vi "AllowEdgeStartCheck.vi"(0 "reference in":refnum<class "UseCaseDiagramGraph.lvclass">, 1 "EdgeStartNode":refnum<class "AbstractNode.lvclass">, 2 "GraphButton":u32, 5 "error in (no error)":errorcluster) -> (14 "reference out":refnum<class "UseCaseDiagramGraph.lvclass">, 16 "Allowed":bool, 19 "error out":errorcluster)   [LabVIEW 2016, in "UseCaseDiagramGraph.lvclass"]
uses:
  <resource>/Framework/Providers/Open_GDS/UML/UseCaseDiagramGraph_class/UseCaseDiagramGraph.lvclass
  <resource>/Framework/Providers/Open_GDS/UML/AbstractNode_class/AbstractNode.lvclass
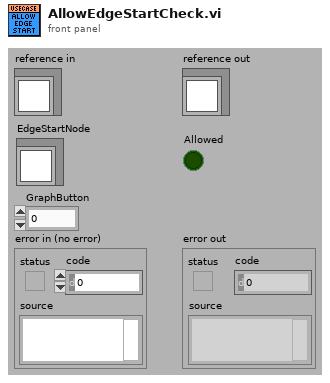
[diagram p1: front panel]
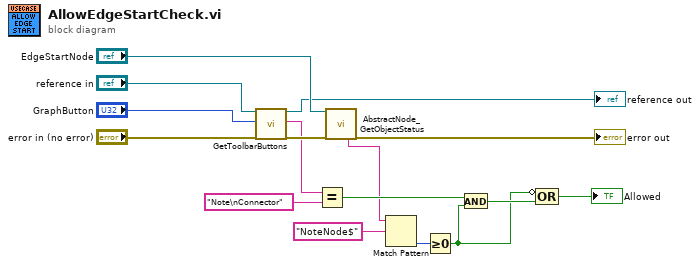
[diagram p0: block diagram]
diagram:
  n1 = call-dynamic "GetToolbarButtons.vi"("reference in"="reference in", "GraphButton"="GraphButton", "error in (no error)"="error in (no error)") -> ("reference out"=→"reference out":refnum<class "UseCaseDiagramGraph.lvclass">, "Text"=w4:string, "error out"=w10:errorcluster)  [unwired: 12 in, 2 out]
  n2 = Equal?(x=w4, y="Note\nConnector" ("Text")) -> (x = y?=w7:bool)
  n3 = call <resource>:"AbstractNode_GetObjectStatus.vi"("reference in"="EdgeStartNode", "error in (no error)"=w10) -> ("Class name"=w6:string, "error out"=→"error out":errorcluster)  [unwired: 16 out]
  n4 = Match Pattern(string=w6, regular expression="NoteNode$") -> (offset past match=w8:i32)  [unwired: 4 out]
  n5 = Greater Or Equal To 0?(x=w8) -> (x >= 0?=w1:bool)
  n6 = And(x=w7, y=w1) -> (x .and. y?=w3:bool)
  n7 = Compound Arithmetic op=OR(invert w1, w3) -> (→"Allowed":bool)
